vi "Week 5_1.vi"() -> ()   [LabVIEW 2015]
uses:
  <vilib>/LabVIEW Interface for Arduino/LabVIEW Interface for Arduino.lvlib
panel:
  in  "VISA resource name":refnum<visa-resource-name>
  in  "stop":bool
  out "Temperature":dbl
  in  "Thermistor AI Pin (0)":u8
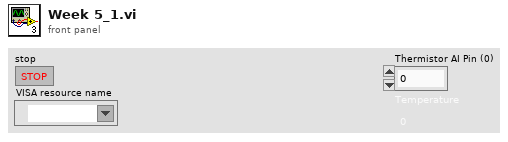
[diagram p1: front panel]
types:
  T1 = typedef "LabVIEW Interface for Arduino.lvlib/Arduino Resource.ctl" = cluster{"VISA resource":refnum<visa-resource-name>, "Board Type":T2, "Connection Type":enum8{"USB / Serial"}, "Bytes Per Packet (15)":u8}
  T2 = typedef "LabVIEW Interface for Arduino.lvlib/Board Type.ctl" = enum16{"Uno", "Dimuelanove w/Atmega 328", "Mega 2560"}
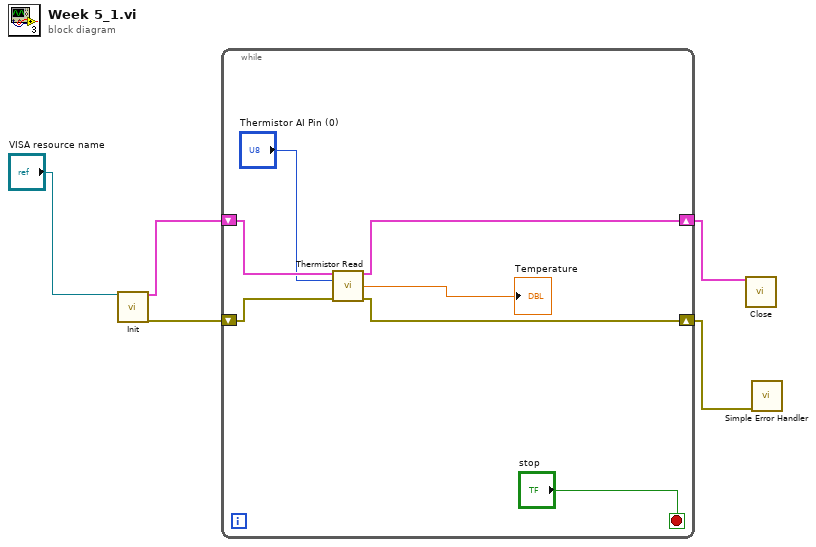
[diagram p0: block diagram]
diagram:
  n1 = call <vilib>:"Init.vi"("VISA resource"="VISA resource name") -> ("Arduino Resource"=w5:T1, "error out"=w4:errorcluster)  [unwired: 17 in]
  n2 = while {
    shift-right: [w9] -> w3
    shift-left: w5 -> [w12]
    shift-right: [w7] -> w2
    shift-left: w4 -> [w11]
    stop <- "stop" stop-if-true
    n3 = call <vilib>:"Thermistor Read.vi"("Arduino Resource"=w12, "Thermistor AI Pin (0)"="Thermistor AI Pin (0)", "error in"=w11) -> ("Arduino Resource"=w9:T1, "Temperature"=→"Temperature":dbl, "error out"=w7:errorcluster)  [unwired: 10 in]
  }
  n4 = call <vilib>:"Close.vi"("Arduino Resource"=w3) -> ()  [unwired: 14 in, 1 out]
  n5 = call <vilib>:"Simple Error Handler.vi"("error in (no error)"=w2) -> ()  [unwired: 4 in, 5 out]
